vi "Translator.Enum.WriteStrings.vi"(8 "error out":errorcluster, 10 "Strings":string[](array[string]), 11 "idx":i32) -> (0 "error out 2":errorcluster)   [LabVIEW 2019, in "Tools.lvlib"]
uses:
  Tools.lvlib
  Translator.Global.vi
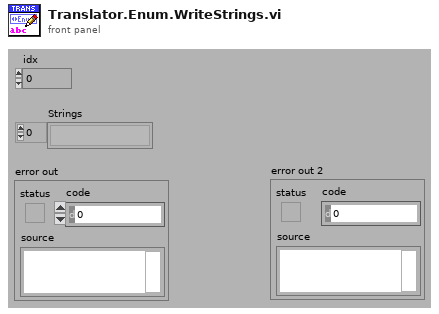
[diagram p1: front panel]
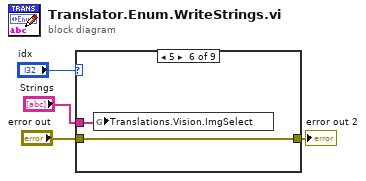
[diagram p0: block diagram]
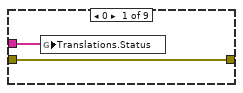
[diagram p2: hidden frame]
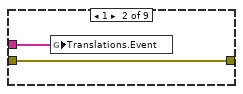
[diagram p3: hidden frame]
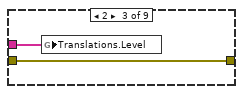
[diagram p4: hidden frame]
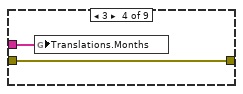
[diagram p5: hidden frame]
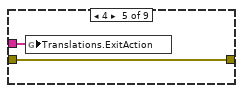
[diagram p6: hidden frame]
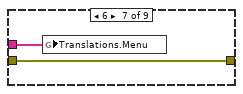
[diagram p7: hidden frame]
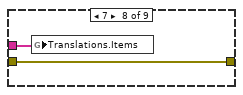
[diagram p8: hidden frame]
diagram:
  n1 = case shown="5" "idx" {
    tunnel: "Strings" -> [w6 w8 w10 w12 w14 w16 w17 w20 _]
    tunnel: "error out" -> [w5 w7 w9 w11 w13 w15 w18 w19 w21]
    tunnel: [w5 w7 w9 w11 w13 w15 w18 w19 w21] -> w2
    frame 0 {
      n2 = global write "Translator.Global.vi" "Translations.Status"(w6) -> ()
    }
    frame 1 {
      n3 = global write "Translator.Global.vi" "Translations.Event"(w8) -> ()
    }
    frame 2 {
      n4 = global write "Translator.Global.vi" "Translations.Level"(w10) -> ()
    }
    frame 3 {
      n5 = global write "Translator.Global.vi" "Translations.Months"(w12) -> ()
    }
    frame 4 {
      n6 = global write "Translator.Global.vi" "Translations.ExitAction"(w14) -> ()
    }
    frame 5 {
      n7 = global write "Translator.Global.vi" "Translations.Vision.ImgSelect"(w16) -> ()
    }
    frame 6 {
      n8 = global write "Translator.Global.vi" "Translations.Menu"(w17) -> ()
    }
    frame 7 {
      n9 = global write "Translator.Global.vi" "Translations.Items"(w20) -> ()
    }
    frame Default {
    }
  }
  "error out 2" <- w2
